vi "ADO Connection Execute.vi"(8 "error in (no error)":errorcluster caption="错误输入（无错误）", 9 "CommandText":string, 10 "cursor type":T1, 11 "Database Connection 输入":refnum<class "Database Connection.lvclass"> caption="DNL_LabVIEW Object in") -> (0 "error out":errorcluster caption="错误输出", 1 "Database Recordset输出":refnum<class "Database Recordset.lvclass">, 3 "Database Connection 输出":refnum<class "Database Connection.lvclass"> caption="DNL_LabVIEW Object out")   [LabVIEW 2011, in "Database Connection.lvclass"]
uses:
  Database Connection.lvclass
  Recordset/Database Recordset.lvclass
  <vilib>/addons/database/Auxilliary.llb/DB Tools Cursor Type.ctl
  Database Connection.lvclass/Database Connection.ctl
  <vilib>/addons/database/NI_Database_API.lvlib
panel:
  in  "ADODB._Recordset":refnum<k7>
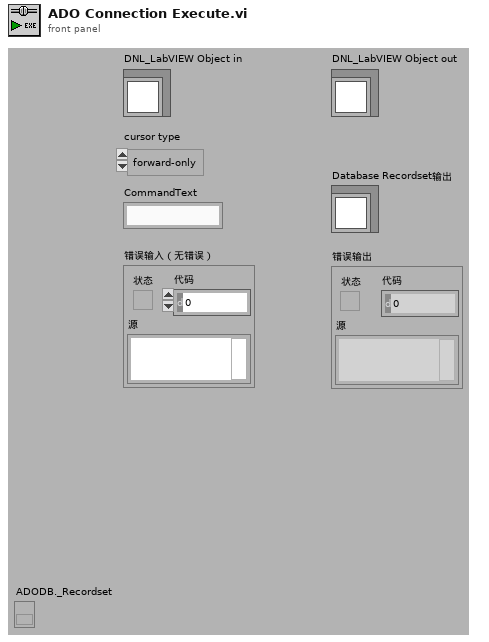
[diagram p1: front panel]
types:
  T1 = typedef "NI_Database_API.lvlib/DB Tools Cursor Type.ctl" = enum16{"forward-only", "keyset", "dynamic", "static"}
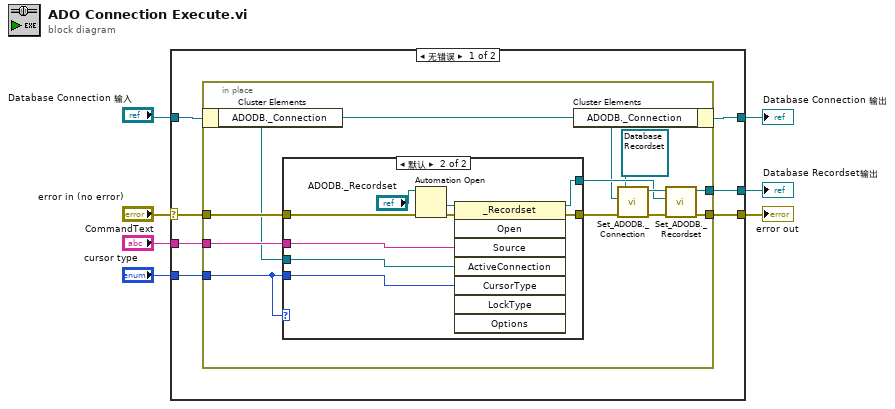
[diagram p0: block diagram]
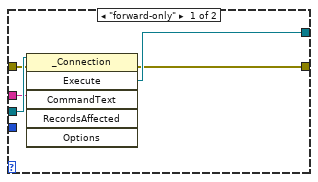
[diagram p2: hidden frame]
diagram:
  n1 = case shown="无错误" "error in (no error)" {
    selector: "error in (no error)" -> [w12 w41]
    tunnel: [w11 w41] -> w6
    tunnel: [w13 w40] -> w4
    tunnel: "Database Connection 输入" -> [w14 w40]
    tunnel: "CommandText" -> [w10 _]
    tunnel: [w9 _] -> w2
    tunnel: "cursor type" -> [w8 _]
    frame No Error {
      n2 = in-place {
        in-place-border: w12 -> [w25]
        in-place-border: [w18] -> w11
        in-place-border: w10 -> [w24]
        in-place-border: [w20] -> w9
        in-place-border: w8 -> [w17]
        n3 = in-place-cluster #1(w14) -> ("ADODB._Connection"=w16:refnum<k7>)
        n4 = case shown="默认" w17 {
          tunnel: w16 -> [w30 w34]
          tunnel: w25 -> [w29 w36]
          tunnel: w24 -> [w28 w35]
          tunnel: [w27 w31] -> w21
          tunnel: [w26 w32] -> w19
          tunnel: w17 -> [_ w33]
          frame "forward-only" {
            n5 = invoke class="_Connection" method="Execute"(reference=w30, error in=w29, "CommandText"=w28) -> (error out=w26:errorcluster, "Execute"=w27:refnum<k7>)  [unwired: 3 in, 4 out]
          }
          frame Default {
            n6 = Automation Open(error in (no error)=w36, Automation Refnum="ADODB._Recordset") -> (Automation Refnum=w38:refnum<k7>, error out=w39:errorcluster)  [unwired: 2 out]
            n7 = invoke class="_Recordset" method="Open"(reference=w38, error in=w39, "Source"=w35, "ActiveConnection"=w34, "CursorType"=w33) -> (reference out=w31:refnum<k7>, error out=w32:errorcluster)  [unwired: 3 in, 6 out]
          }
        }
        n8 = in-place-cluster #1("ADODB._Connection"=w16) -> (w13:refnum<class "Database Connection.lvclass">)
        n9 = call "Set_ADODB._Connection.vi"("error in (no error)"=w19, "ADODB._Connection"=w16, "Database Recordset输入"=refnum<class "Database Recordset.lvclass"> refnum ("Database Recordset.lvclass")) -> ("error out"=w22:errorcluster, "Database Recordset输出"=w23:refnum<class "Database Recordset.lvclass">)  [unwired: 7 in]
        n10 = call "Set_ADODB._Recordset.vi"("error in (no error)"=w22, "ADODB._Recordset"=w21, "Database Recordset输入"=w23) -> ("error out"=w18:errorcluster, "Database Recordset输出"=w20:refnum<class "Database Recordset.lvclass">)  [unwired: 7 in]
      }
    }
    frame Error {
    }
  }
  "error out" <- w6
  "Database Connection 输出" <- w4
  "Database Recordset输出" <- w2
